vi "Seriala.vi"() -> ()   [LabVIEW 2020]
uses:
  <vilib>/Instr/_visa.llb/VISA Configure Serial Port (Instr).vi
panel:
  out "Waveform Chart":cluster{i32, i32}(graph)
  out "read buffer":string
  in  "stop":bool
  in  "Bluetooth":refnum<visa-resource-name>="COM7"
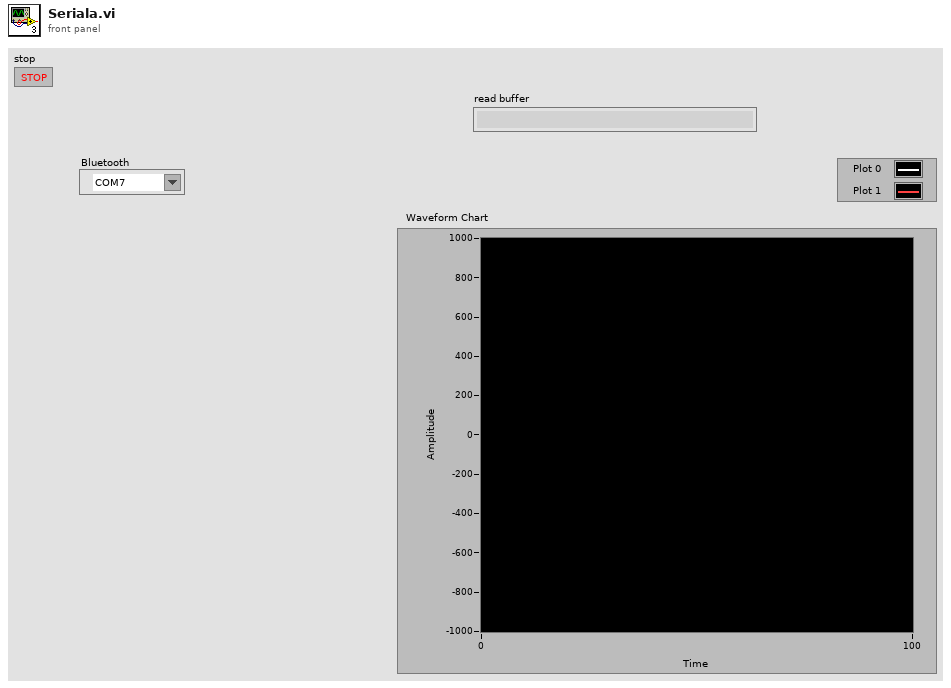
[diagram p1: front panel]
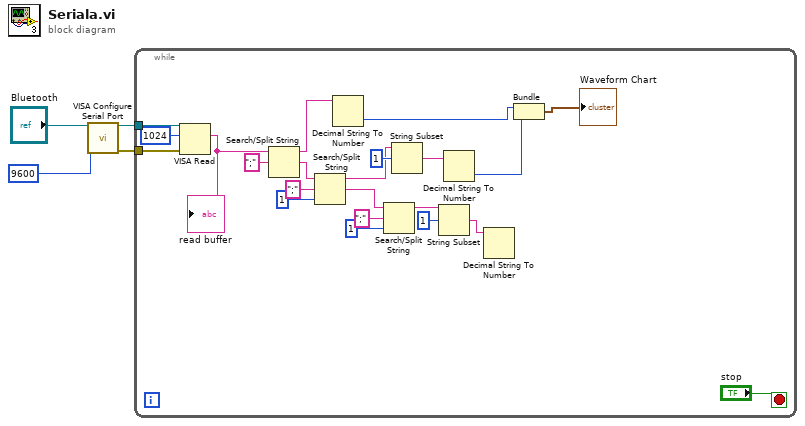
[diagram p0: block diagram]
diagram:
  n1 = call-poly "VISA Configure Serial Port"("VISA resource name"="Bluetooth", "baud rate (9600)"=u32 9600) -> ("VISA resource name out"=w1:refnum<visa-resource-name>, "error out"=w2:errorcluster)  [unwired: 12 in]
  n2 = while {
    tunnel: w2 -> [w26]
    tunnel: w1 -> [w25]
    stop <- "stop" stop-if-true
    n3 = VISA Read(VISA resource name=w25, byte count=u32 1024, error in (no error)=w26) -> (read buffer=w22:string)  [unwired: 3 out]
    "read buffer" <- w22
    n4 = Search/Split String(string=w22, search string/char (-)=";") -> (substring before match=w12:string, match + rest of string=w20:string)  [unwired: 1 in, 1 out]
    n5 = Search/Split String(string=w20, search string/char (-)=";", offset (0)=1) -> (substring before match=w11:string, match + rest of string=w15:string)  [unwired: 1 out]
    n6 = Decimal String To Number(string=w12) -> (number=w7:i32)  [unwired: 2 in, 1 out]
    n7 = Search/Split String(string=w15, search string/char (-)=";", offset (0)=1) -> (substring before match=w10:string)  [unwired: 2 out]
    n8 = String Subset(string=w11, offset (0)=1) -> (substring=w9:string)  [unwired: 1 in]
    n9 = String Subset(string=w10, offset (0)=1) -> (substring=w8:string)  [unwired: 1 in]
    n10 = Decimal String To Number(string=w9) -> (number=w6:i32)  [unwired: 2 in, 1 out]
    n11 = Decimal String To Number(string=w8) -> ()  [unwired: 2 in, 2 out]
    n12 = Bundle(w7, w6) -> (→"Waveform Chart":cluster{i32, i32})  [unwired: 1 in]
  }
